vi "Read Class Instance.vi"(8 "error in (no error)":errorcluster, 11 "Test Runner.Project in":refnum<class "Test Runner.Class.lvclass">) -> (0 "error out":errorcluster, 2 "Instance":refnum<class>, 3 "Test Runner.Project out":refnum<class "Test Runner.Class.lvclass">)   [LabVIEW 2013, in "Caraya.lvlib" / "Test Runner.Class.lvclass"]
uses:
  Test Runner.Class.lvclass
  Test Runner.Class.lvclass/Test Runner.Class.ctl
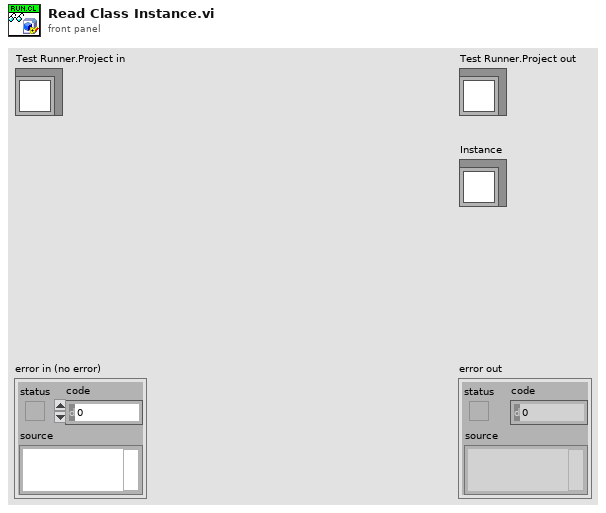
[diagram p1: front panel]
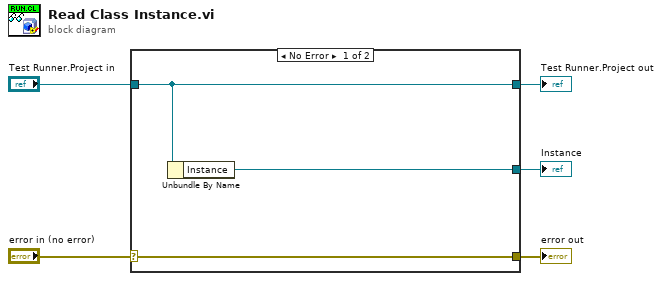
[diagram p0: block diagram]
diagram:
  n1 = case shown="No Error" "error in (no error)" {
    selector: "error in (no error)" -> [w8 w9]
    tunnel: [w8 w9] -> w4
    tunnel: [w7 w10] -> w2
    tunnel: "Test Runner.Project in" -> [w7 w10]
    tunnel: [w6 _] -> w1
    frame No Error {
      n2 = Unbundle By Name(w7) -> ("Instance"=w6:refnum<class>)
    }
    frame Error {
    }
  }
  "error out" <- w4
  "Test Runner.Project out" <- w2
  "Instance" <- w1
